vi "Soft Panel.vi"(8 "error in (no error)":errorcluster, 11 "JMETestSolutions.Instrument.DMM in":refnum<class "JMETestSolutions.Instrument.DMM.lvclass">) -> (0 "error out":errorcluster, 3 "JMETestSolutions.Instrument.DMM out":refnum<class "JMETestSolutions.Instrument.DMM.lvclass">)   [LabVIEW 2020, in "JMETestSolutions.Instrument.DMM.lvlib" / "JMETestSolutions.Instrument.DMM.lvclass"]
uses:
  JMETestSolutions.Instrument.DMM.lvclass
panel:
  in  "stop":bool
  # "DMM Soft Panel"
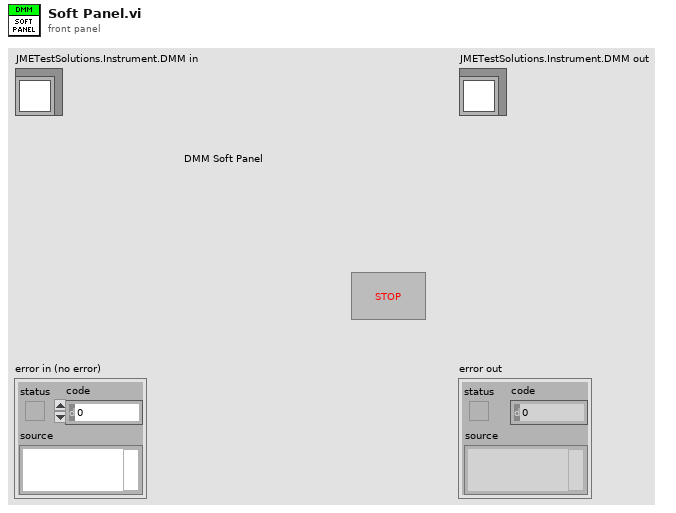
[diagram p1: front panel]
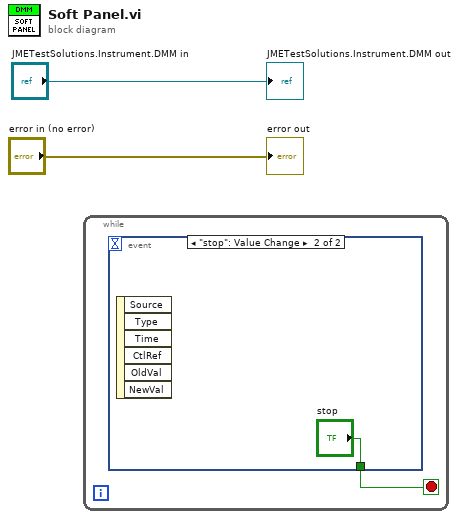
[diagram p0: block diagram]
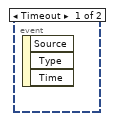
[diagram p2: hidden frame]
diagram:
  n1 = while {
    stop <- w3 stop-if-true
    n2 = event shown="[1] \"stop\": Value Change" {
      selector: _ -> [_ _]
      dyn-events: _ -> [_ _]
      timeout: _ -> [_ _]
      tunnel: [_ "stop"] -> w3
      event Timeout {
        n3 = event-data() -> ()  [unwired: 1 in, 3 out]
      }
      event "stop": Value Change {
        n4 = event-data() -> ()  [unwired: 1 in, 6 out]
      }
    }
  }
  "error out" <- "error in (no error)"
  "JMETestSolutions.Instrument.DMM out" <- "JMETestSolutions.Instrument.DMM in"
